vi "Subset (single).vi"(8 "error in (no error)":errorcluster, 9 "Subset Method":enum16{"Slider (%)", "X[] min and max"}(ring)=enum."X[] min and max", 10 "Subset Slider (%)":cluster{dbl, dbl}(slide)={75.0, 25.0} scale=0.0..100.0 scale format="%#_6f", 11 "XY-data":cluster{"X-array":dbl[], "Y-array":dbl[]}) -> (0 "error out":errorcluster, 3 "XY-data out":cluster{"X-array":dbl[], "Y-array":dbl[]} {"Y-array" format="%.2p"; "X-array" format="%.2p"})   [LabVIEW 2016, in "xy_utilities.lvlib"]
doc: "Returns a subset of <b>XY-data</b>\n\n<b>Subset Method</b>: choose how to define the subset.\n- <b>X[] min and max</b>: returns subset of data between found maximum and minimum values of <b>x-array</b>. Returns data in ascending x order.\n- Slider: chooses data subset based on percentages (%) defined by <b>Subset Slider</b> \n\nWire data to the data input to determine the polymorphic instance to use or manually select the instance."
uses:
  xy_utilities.lvlib
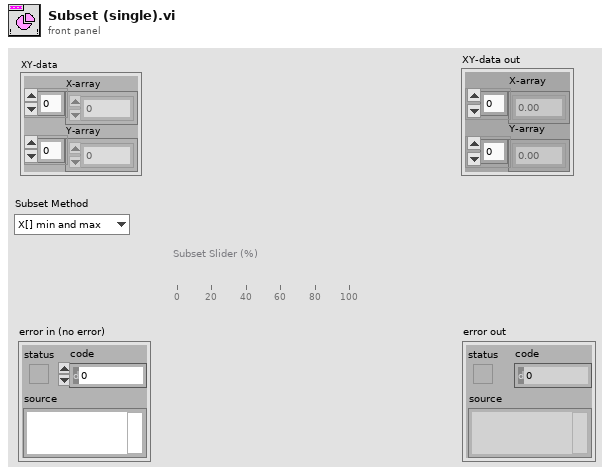
[diagram p1: front panel]
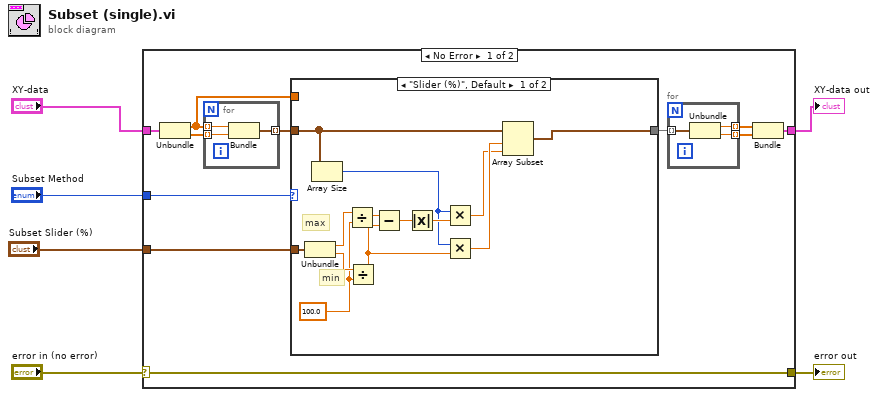
[diagram p0: block diagram]
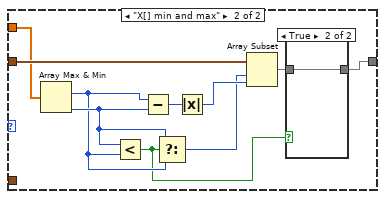
[diagram p2: hidden frame]
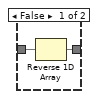
[diagram p3: hidden frame]
diagram:
  n1 = case shown="No Error" "error in (no error)" {
    selector: "error in (no error)" -> [w17 w51]
    tunnel: [w17 w51] -> w6
    tunnel: "XY-data" -> [w16 w50]
    tunnel: [w9 w50] -> w5
    tunnel: "Subset Method" -> [w13 _]
    tunnel: "Subset Slider (%)" -> [w8 _]
    frame No Error {
      n2 = Unbundle(w16) -> ("X-array"=w7:dbl[], "Y-array"=w15:dbl[])
      n3 = for {
        tunnel: w7 -> [w49] mode=indexing
        tunnel: w15 -> [w48] mode=indexing
        tunnel: [w47] -> w14 mode=indexing
        n4 = Bundle("x"=w49, "y"=w48) -> (w47:cluster{"x":dbl, "y":dbl})  [unwired: 1 in]
      }
      n5 = case shown="\"Slider (%)\", Default" w13 {
        tunnel: w14 -> [w27 w41]
        tunnel: [w26 w35] -> w10
        tunnel: w8 -> [w24 _]
        tunnel: w7 -> [_ w40]
        frame "Slider (%)", Default {
          w21 = 100.0 ("y")
          # "min"
          # "max"
          n6 = Unbundle(w24) -> (w28:dbl, w25:dbl)
          n7 = Array Size(array=w27) -> (size(s)=w30:i32)
          n8 = Divide(x=w28, y=w21) -> (x/y=w22:dbl)
          n9 = Divide(x=w25, y=w21) -> (x/y=w23:dbl)
          n10 = Subtract(x=w22, y=w23) -> (x-y=w29:dbl)
          n11 = Absolute Value(x=w29) -> (abs(x)=w31:dbl)
          n12 = Multiply(x=w30, y=w31) -> (x*y=w32:dbl)
          n13 = Multiply(x=w30, y=w23) -> (x*y=w33:dbl)
          n14 = Array Subset(array=w27, index=w33, length=w32) -> (w26:cluster{"x":dbl, "y":dbl}[])
        }
        frame "X[] min and max" {
          n15 = Array Max & Min(array=w40) -> (max index (indices)=w37:i32, min index (indices)=w38:i32)  [unwired: 2 out]
          n16 = Less?(x=w38, y=w37) -> (x < y?=w34:bool)
          n17 = Subtract(x=w37, y=w38) -> (x-y=w42:i32)
          n18 = Select(t=w38, s=w34, f=w37) -> (s? t:f=w36:i32)
          n19 = Absolute Value(x=w42) -> (abs(x)=w43:i32)
          n20 = Array Subset(array=w41, index=w36, length=w43) -> (w39:cluster{"x":dbl, "y":dbl}[])
          n21 = case shown="True" w34 {
            tunnel: w39 -> [w45 w46]
            tunnel: [w44 w46] -> w35
            frame False {
              n22 = Reverse 1D Array(array=w45) -> (reversed array=w44:cluster{"x":dbl, "y":dbl}[])
            }
            frame True {
            }
          }
        }
      }
      n23 = for {
        tunnel: w10 -> [w20] mode=indexing
        tunnel: [w19] -> w11 mode=indexing
        tunnel: [w18] -> w12 mode=indexing
        n24 = Unbundle(w20) -> ("x"=w19:dbl, "y"=w18:dbl)
      }
      n25 = Bundle(w11, w12) -> (w9:cluster{dbl[], dbl[]})  [unwired: 1 in]
    }
    frame Error {
    }
  }
  "error out" <- w6
  "XY-data out" <- w5
